vi "Custom Command Template.vi"(8 "Error In":errorcluster, 11 "LINX Resource":T1) -> (0 "Error Out":errorcluster, 3 "LINX Resource":T1)   [LabVIEW 2011, in "LVH-LINX.lvlib"]
uses:
  LVH-LINX.lvlib
  Private/Type Defs/LINX Ref.ctl
  Private/Type Defs/Platform.ctl
  Private/Type Defs/Interface.ctl
  Private/Device/Type Defs/LINX Device Config.ctl
  Private/Device/Type Defs/TCP Config.ctl
  Private/Device/Type Defs/Channels.ctl
  Private/Type Defs/Error Type.ctl
  Private/Device/Device.lvlib
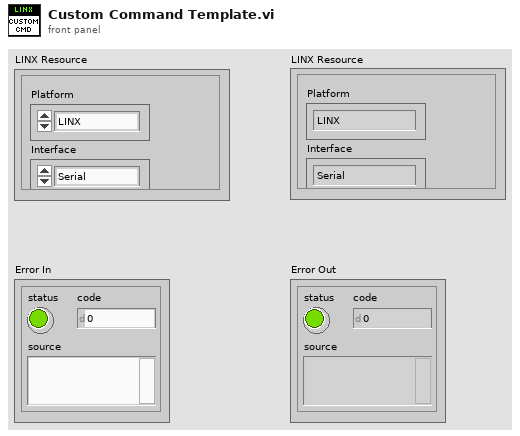
[diagram p1: front panel]
types:
  T1 = typedef "LVH-LINX.lvlib/LINX Ref.ctl" = cluster{"Platform":T2, "Interface":T3, "LINX Device Config":T4}
  T2 = typedef "LVH-LINX.lvlib/Platform.ctl" = enum16{"LINX", "myRIO"}
  T3 = typedef "LVH-LINX.lvlib/Interface.ctl" = enum16{"Serial", "TCP"}
  T4 = typedef "LVH-LINX.lvlib/Device.lvlib/LINX Device Config.ctl" = cluster{"Interface":T3, "COM Port":refnum<visa-resource-name>, "TCP Configuration":T5, "Device Family":u8, "Device ID":u8, "Device Name":string, "TCP Ref":refnum<k5>, "Channels":T6}
  T5 = typedef "LVH-LINX.lvlib/Device.lvlib/TCP Config.ctl" = cluster{"IP Address":string, "Port":u16}
  T6 = typedef "LVH-LINX.lvlib/Channels.ctl" = cluster{"DI Channels":u8[], "DO Channels":u8[], "AI":u8[], "AO":u8[], "PWM":u8[], "QE":u8[], "UART":u8[], "I2C 2":u8[], "SPI":u8[], "CAN":u8[], "AI Ref (V)":dbl, "AO Resolution (Bits)":u8, "AO Ref (V)":dbl}
  T7 = typedef "LVH-LINX.lvlib/Error Type.ctl" = enum16{"Unknown", "Timeout", "Corrupt Return Packet", "Unable To Connect", "Command Not Supported", "Channel DNE", "Invalid COM Config", "Firmware Version Mismatch", "myRIO Support"}
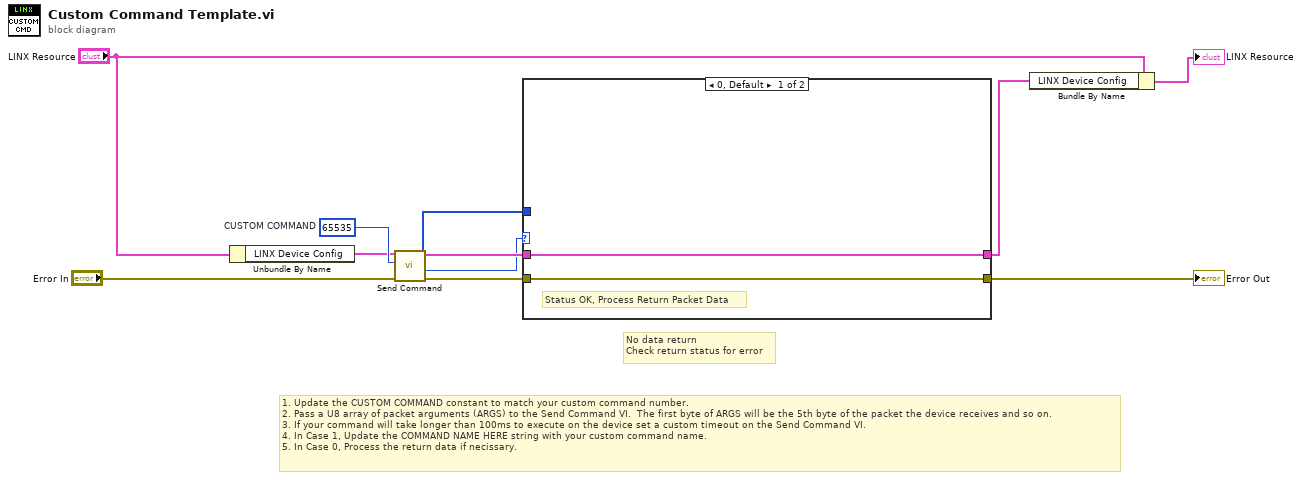
[diagram p0: block diagram]
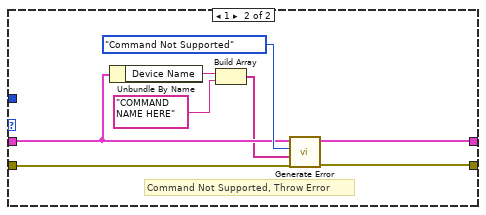
[diagram p2: hidden frame]
diagram:
  w9 = u16 65535  # CUSTOM COMMAND
  # "1. Update the CUSTOM COMMAND constant to match your custom command number.\n2. Pass a U8 array of packet arguments (ARGS) to the Send Command VI.  The first byte of ARGS will be the 5th byte of the packet the device receives and so on.\n3. If your command will take longer than 100ms to execute on the device set a custom timeout on the Send Command VI.\n4. In Case 1, Update the COMMAND NAME HERE string with your custom command name.\n5. In Case 0, Process the return data if necissary."
  # "No data return\nCheck return status for error"
  n1 = Unbundle By Name("LINX Resource") -> ("LINX Device Config"=w3:T4)
  n2 = call "Send Command.vi"("Error In"="Error In", "CMD"=w9, "LINX Device Config"=w3) -> ("Error Out"=w6:errorcluster, "Status"=w1:u8, "Response"=w5:u8[], "LINX Device Config"=w8:T4)  [unwired: 5 in]
  n3 = case shown="0, Default" w1 {
    tunnel: [w13 w19] -> w4
    tunnel: w8 -> [w13 w15]
    tunnel: [w12 w20] -> w7
    tunnel: w6 -> [w12 w21]
    tunnel: w5 -> [_ _]
    frame 0, Default {
      # "Status OK, Process Return Packet Data"
    }
    frame 1 {
      # "Command Not Supported, Throw Error"
      n4 = Unbundle By Name(w15) -> ("Device Name"=w17:string)
      n5 = Build Array(w17, "COMMAND NAME HERE") -> (w14:string[])
      n6 = call "Generate Error.vi"("Error In"=w21, "Arguments"=w14, "Error Type"=Error_Type."Command Not Supported", "LINX Device Config"=w15) -> ("Error Out"=w20:errorcluster, "LINX Device Config"=w19:T4)  [unwired: 6 in]
    }
  }
  "Error Out" <- w7
  n7 = Bundle By Name(cluster="LINX Resource", "LINX Device Config"=w4) -> (→"LINX Resource":T1)
